vi "单控 慢速到液位命令.vi"(7 "是否启用通讯通知":bool, 8 "error in (no error)":errorcluster, 10 "慢速到液位":bool, 11 "Slave ID":T1) -> (0 "error out":errorcluster)   [LabVIEW 2016, in "质控单元V1.lvlib"]
uses:
  <vilib>/Plasmionique/MB Master/MB_Master/MB_Master.lvclass
  <vilib>/Plasmionique/MB Master/MB Master.lvlib
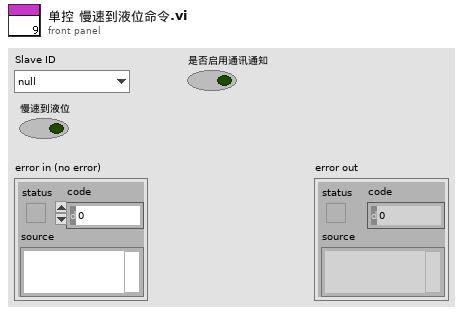
[diagram p1: front panel]
types:
  T1 = typedef "质控单元V1.lvlib/质控slave id.ctl" = enum16{"null", "氨氮", "总磷", "CODMn", "CODCr", "总氮"}
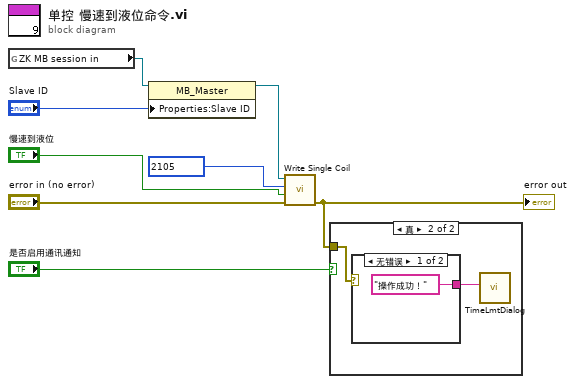
[diagram p0: block diagram]
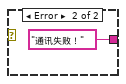
[diagram p3: hidden frame]
diagram:
  n1 = global read "ZK非断电保存全局变量.vi" "ZK MB session in"() -> (w7:refnum<class "MB_Master.lvclass">)
  n2 = property class="MB_Master"(reference=w7, "Properties:Slave ID"="Slave ID") -> (reference out=w5:refnum<class "MB_Master.lvclass">)  [unwired: 1 in, 1 out]
  n3 = call <vilib>:"Write Single Coil.vi"("error in (no error)"="error in (no error)", "value"="慢速到液位", "address"=u16 2105 ("starting address"), "MB session in"=w5) -> ("error out"=w2:errorcluster)  [unwired: 6 in, 1 out]
  "error out" <- w2
  n4 = case shown="真" "是否启用通讯通知" {
    tunnel: w2 -> [_ w10]
    frame False {
    }
    frame True {
      n5 = case shown="无错误" w10 {
        tunnel: ["操作成功！" "通讯失败！"] -> w9
        frame No Error {
        }
        frame Error {
        }
      }
      n6 = call "TimeLmtDialog.vi"("Infoin"=w9) -> ()  [unwired: 11 in]
    }
  }
